vi "PRO_VerifySpecV1.vi"(6 "error in (no error)":errorcluster, 7 "Enable":bool, 8 "Results in":T7=[[{"Fill"=0.0, "Drain"=7.150000000000002, "Status"=9, "Resistor"=100.0}, {"Fill"=0.0, "Drain"=6.925000000000003, "Status"=9, "Resistor"=100.0}], [{"Fill"=7.1350000000000025, "Drain"=6.700000000000004, "Status"=9, "Resistor"=200.0}, {"Fill"=6.910000000000004, "Drain"=6.475000000000005, "Status"=9, "Resistor"=200.0}], [{"Fill"=6.685000000000004, "Drain"=6.250000000000005, "Status"=9, "Resistor"=300.0}, {"Fill"=6.460000000000004, "Drain"=6.025000000000006, "Status"=9, "Resistor"=300.0}], [{"Fill"=6.235000000000006, "Drain"=5.8000000000000025, "Status"=9, "Resistor"=400.0}, {"Fill"=6.010000000000005, "Drain"=5.59, "Status"=9, "Resistor"=400.0}], [{"Fill"=5.785000000000002, "Drain"=5.364999999999997, "Status"=9, "Resistor"=500.0}, {"Fill"=5.574999999999999, "Drain"=5.1399999999999935, "Status"=9, "Resistor"=500.0}], [{"Fill"=5.349999999999996, "Drain"=4.91499999999999, "Status"=9, "Resistor"=600.0}, {"Fill"=5.124999999999993, "Drain"=4.689999999999987, "Status"=9, "Resistor"=600.0}], [{"Fill"=4.89999999999999, "Drain"=4.464999999999983, "Status"=9, "Resistor"=700.0}, {"Fill"=4.6749999999999865, "Drain"=4.23999999999998, "Status"=9, "Resistor"=700.0}], [{"Fill"=4.449999999999983, "Drain"=4.014999999999977, "Status"=9, "Resistor"=800.0}, {"Fill"=4.22499999999998, "Drain"=3.7899999999999734, "Status"=9, "Resistor"=800.0}], [{"Fill"=3.999999999999977, "Drain"=3.56499999999997, "Status"=9, "Resistor"=900.0}, {"Fill"=3.7749999999999737, "Drain"=3.339999999999967, "Status"=9, "Resistor"=900.0}], [{"Fill"=3.5499999999999705, "Drain"=3.114999999999964, "Status"=9, "Resistor"=1000.0}, {"Fill"=3.3249999999999673, "Drain"=2.8899999999999606, "Status"=9, "Resistor"=1000.0}], [{"Fill"=3.099999999999964, "Drain"=0.0, "Status"=5, "Resistor"=1100.0}, {"Fill"=2.874999999999961, "Drain"=0.0, "Status"=5, "Resistor"=1100.0}]] {"Resistor" format="%.1f"; "Drain" format="%.3f"; "Fill" format="%.3f"}, 9 "Measure In":T6={"Ch A   Ohms"=100.0, " Ch B  Ohms"=100.0, "Level OUt"=3.672222222222213}, 10 "Specs In":T1, 11 "Switched In":bool[](array[boolean])) -> (0 "Results out":T7=[[{"Fill"=0.0, "Drain"=7.150000000000002, "Status"=9, "Resistor"=100.0}, {"Fill"=0.0, "Drain"=6.925000000000003, "Status"=9, "Resistor"=100.0}], [{"Fill"=7.1350000000000025, "Drain"=6.700000000000004, "Status"=9, "Resistor"=200.0}, {"Fill"=6.910000000000004, "Drain"=6.475000000000005, "Status"=9, "Resistor"=200.0}], [{"Fill"=6.685000000000004, "Drain"=6.250000000000005, "Status"=9, "Resistor"=300.0}, {"Fill"=6.460000000000004, "Drain"=6.025000000000006, "Status"=9, "Resistor"=300.0}], [{"Fill"=6.235000000000006, "Drain"=5.8000000000000025, "Status"=9, "Resistor"=400.0}, {"Fill"=6.010000000000005, "Drain"=5.59, "Status"=9, "Resistor"=400.0}], [{"Fill"=5.785000000000002, "Drain"=5.364999999999997, "Status"=9, "Resistor"=500.0}, {"Fill"=5.574999999999999, "Drain"=5.1399999999999935, "Status"=9, "Resistor"=500.0}], [{"Fill"=5.349999999999996, "Drain"=4.91499999999999, "Status"=9, "Resistor"=600.0}, {"Fill"=5.124999999999993, "Drain"=4.689999999999987, "Status"=9, "Resistor"=600.0}], [{"Fill"=4.89999999999999, "Drain"=4.464999999999983, "Status"=9, "Resistor"=700.0}, {"Fill"=4.6749999999999865, "Drain"=4.23999999999998, "Status"=9, "Resistor"=700.0}], [{"Fill"=4.449999999999983, "Drain"=4.014999999999977, "Status"=9, "Resistor"=800.0}, {"Fill"=4.22499999999998, "Drain"=3.7899999999999734, "Status"=9, "Resistor"=800.0}], [{"Fill"=3.999999999999977, "Drain"=3.56499999999997, "Status"=9, "Resistor"=900.0}, {"Fill"=3.7749999999999737, "Drain"=3.339999999999967, "Status"=9, "Resistor"=900.0}], [{"Fill"=3.5499999999999705, "Drain"=3.114999999999964, "Status"=9, "Resistor"=1000.0}, {"Fill"=3.3249999999999673, "Drain"=2.8899999999999606, "Status"=9, "Resistor"=1000.0}], [{"Fill"=3.099999999999964, "Drain"=0.0, "Status"=5, "Resistor"=1100.0}, {"Fill"=2.874999999999961, "Drain"=0.0, "Status"=5, "Resistor"=1100.0}]] {"Resistor" format="%.1f"; "Drain" format="%.3f"; "Fill" format="%.3f"}, 1 "Status Code":i32, 3 "Switched Out":bool[](array[boolean]), 4 "error out":errorcluster)   [LabVIEW 2024]
doc: "Compares the ChA, ChB and Level measurements to the Incexed Spec Row. Checks for R Switch Value occured in Switch Zone, The resistor level was consistand in the In Range Zone, and records the R level in ohms at the R measurement point. \n\nBuilds the Results Table."
uses:
  Control Definitions/Def Results2.ctl
  Control Definitions/Ded LUT_Status.ctl
  Control Definitions/Def PumpCtlRefs.ctl
  Control Definitions/DEF_SpecsOut.ctl
  Control Definitions/Def_ATPStatus.ctl
  Control Definitions/Def_PumpSpeed.ctl
  Control Definitions/Def Spec RNG.ctl
  Control Definitions/Def TestState.ctl
panel:
  # "ChA=0; ChB=1"
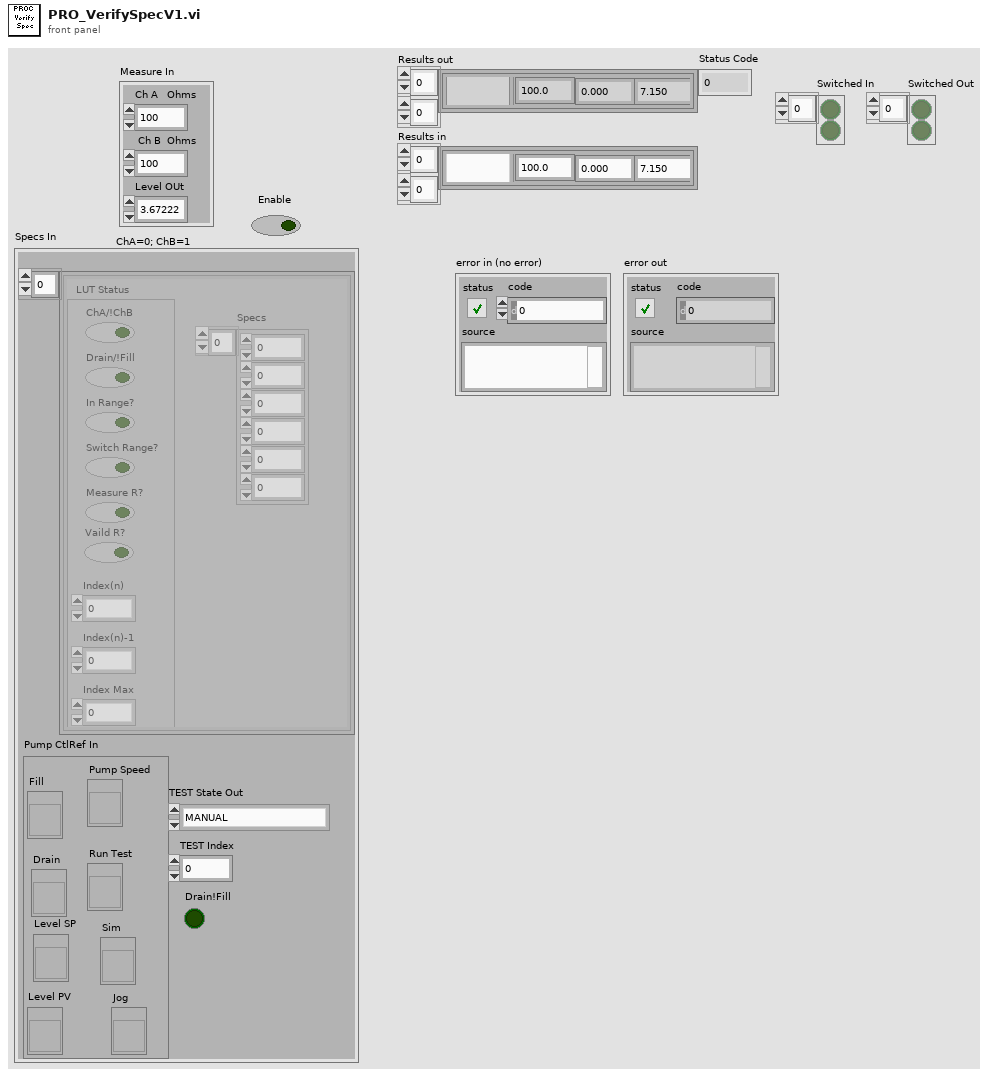
[diagram p1: front panel]
types:
  T1 = typedef "DEF_SpecsOut.ctl" = cluster{"aSpecsTable":T2[], "Pump CtlRef In":T4, "TEST State Out":T5, "TEST Index":i32, "Drain!Fill":bool}
  T2 = typedef "Def Spec RNG.ctl" = cluster{"Specs":dbl[], "LUT Status":T3}
  T3 = typedef "Ded LUT_Status.ctl" = cluster{"ChA/!ChB":bool, "Drain/!Fill":bool, "In Range?":bool, "Switch Range?":bool, "Measure R?":bool, "Vaild R?":bool, "Index(n)":i32, "Index(n)-1":i32, "Index Max":i32, "Index(n-1)":i32}
  T4 = typedef "Def PumpCtlRefs.ctl" = cluster{"Fill ":refnum<vi>, "Drain":refnum<vi>, "Level PV":refnum<vi>, "Pump Speed":refnum<vi>, "Run Test":refnum<vi>, "Sim":refnum<vi>, "Jog":refnum<vi>, "Level SP":refnum<vi>}
  T5 = typedef "Def TestState.ctl" = enum16{"MANUAL", "Start", "Pre-Fill", "Pre-Fill Measure", "Pre-Drain", "Pre-Drin Measure", "Init-Record", "Load Fill Spec", "Filling Hi", "Wait1", "Record Fill", "Load Drain Spec", "Draining Lo", "Wait2", "Record Drain", "Empty", "Done"}
  T6 = cluster{"Ch A   Ohms":dbl, " Ch B  Ohms":dbl, "Level OUt":dbl}
  T7 = typedef "Def Results2.ctl" = cluster{"Fill":dbl, "Drain":dbl, "Status":T8, "Resistor":dbl}[][]
  T8 = typedef "Def_ATPStatus.ctl" = i16
  T9 = cluster{"Fill":dbl, "Drain":dbl, "Status":T8, "Resistor":dbl}
  T10 = cluster{"Fill":dbl, "Drain":dbl, "Status":i16, "Resistor":dbl}[]
  T11 = typedef "Def_LevelSwitched.ctl" = cluster{"Switched":bool, "Level OUt":dbl, "Double Err":bool}
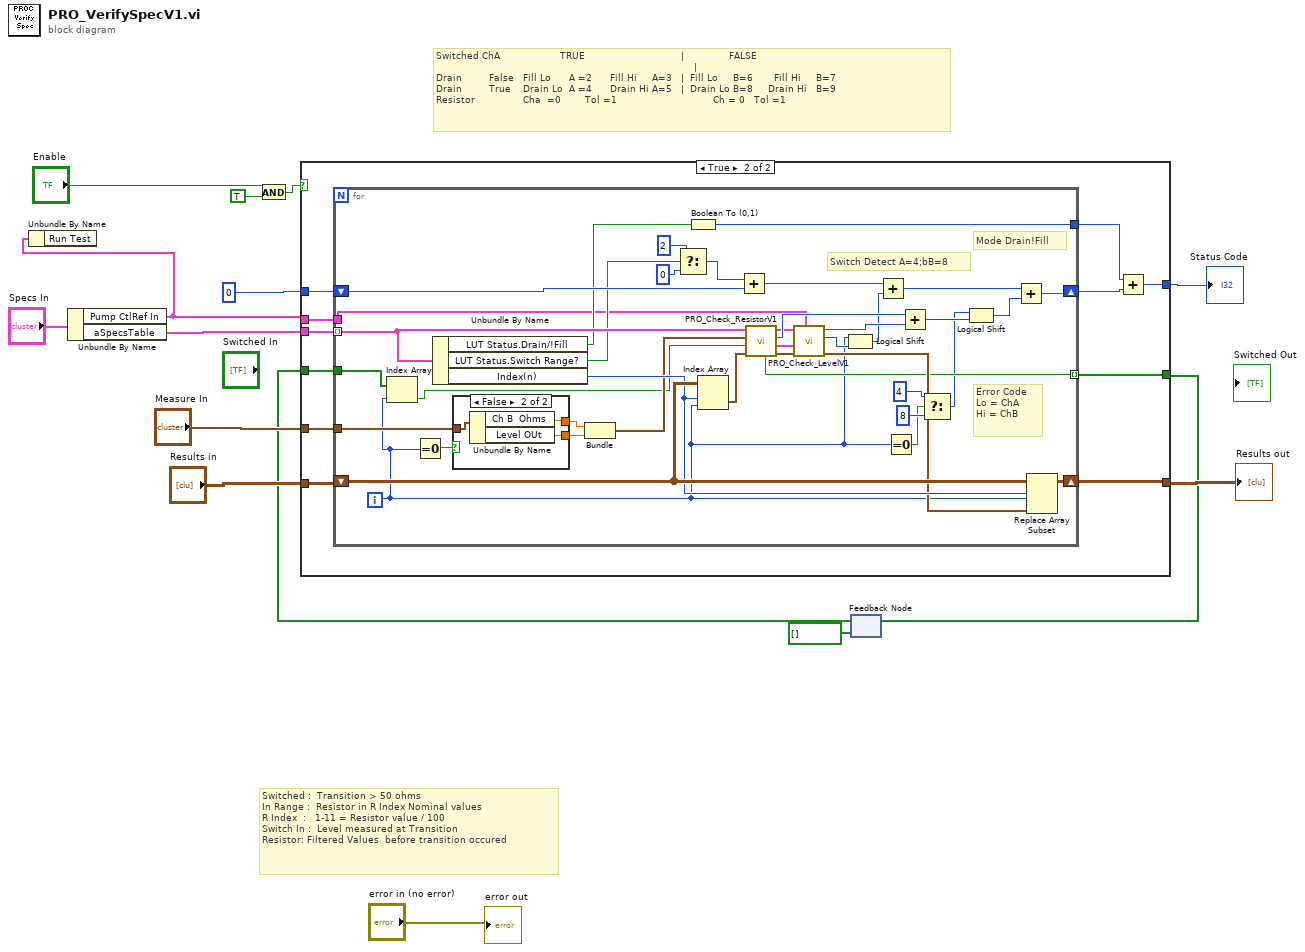
[diagram p0: block diagram]
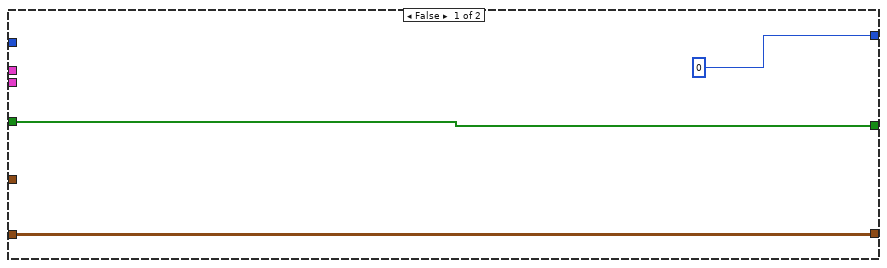
[diagram p2: hidden frame]
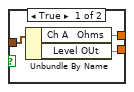
[diagram p3: hidden frame]
diagram:
  # "Switched ChA                    TRUE                                |               FALSE\n                                                                                      |\nDrain         False   Fill Lo      A =2      Fill Hi     A=3   |  Fill Lo     B=6       Fill Hi     B=7\nDrain         True    Drain Lo  A =4      Drain Hi A=5   |  Drain Lo B=8     Drain Hi   B=9 \nResistor                Cha  =0        Tol =1                                Ch = 0   Tol =1"
  # "Switched :  Transition > 50 ohms\nIn Range :  Resistor in R Index Nominal values\nR Index  :   1-11 = Resistor value / 100\nSwitch In :  Level measured at Transition\nResistor: Filtered Values  before transition occured"
  n1 = Unbundle By Name("Specs In") -> ("Pump CtlRef In"=w7:T4, "aSpecsTable"=w8:T2[])
  n2 = Unbundle By Name(w7) -> ()  [unwired: 1 out]
  n3 = And(x="Enable", y=TRUE) -> (x .and. y?=w6:bool)
  n4 = feedback #1(bool[] []) -> (w3:bool[])
  n5 = case shown="True" w6 {
    tunnel: w8 -> [_ w29]
    tunnel: "Results in" -> [w17 w28]
    tunnel: [w17 w27] -> w13
    tunnel: 0 -> [_ w26]
    tunnel: [0 w22] -> w11
    tunnel: "Measure In" -> [_ w25]
    tunnel: w3 -> [w16 w23]
    tunnel: [w16 w24] -> w4
    tunnel: w7 -> [_ w19]
    frame False {
    }
    frame True {
      n6 = for {
        tunnel: w29 -> [w62] mode=indexing
        shift-right: [w52] -> w27
        shift-left: w28 -> [w68]
        shift-right: [w49] -> w21
        shift-left: w26 -> [w43]
        tunnel: w25 -> [w65]
        tunnel: [w51] -> w24 mode=indexing
        tunnel: w23 -> [w55]
        tunnel: [w34] -> w20
        tunnel: w19 -> [w30]
        i -> [w40]
        # "Switch Detect A=4;bB=8"
        # "Mode Drain!Fill"
        # "Error Code\nLo = ChA\nHi = ChB"
        n7 = Index Array(array=w55, index=w40) -> (element=w31:bool)
        n8 = Equal To 0?(x=w40) -> (x = 0?=w64:bool)
        n9 = Unbundle By Name(w62) -> ("LUT Status.Drain/!Fill"=w36:bool, "LUT Status.Switch Range?"=w33:bool, "Index(n)"=w67:i32)
        n10 = case shown="False" w64 {
          tunnel: w65 -> [w71 w74]
          tunnel: [w70 w73] -> w63
          tunnel: [w69 w72] -> w32
          frame True {
            n11 = Unbundle By Name(w71) -> ("Ch A   Ohms"=w70:dbl, "Level OUt"=w69:dbl)
          }
          frame False {
            n12 = Unbundle By Name(w74) -> ("Ch B  Ohms"=w73:dbl, "Level OUt"=w72:dbl)
          }
        }
        n13 = Bundle("Ch B  Ohms"=w63, "Level OUt"=w32) -> (w61:cluster{" Ch B  Ohms":dbl, "Level OUt":dbl})  [unwired: 1 in]
        n14 = Select(t=2, s=w33, f=0) -> (s? t:f=w35:i32)
        n15 = Boolean To (0,1)(Boolean=w36) -> (0, 1=w34:i16)
        n16 = Index Array(array=w68, index (row)=w67, index (col)=w40) -> (element=w60:T9)
        n17 = Add(x=w35, y=w43) -> (x+y=w42:i32)
        n18 = call "PRO_Check_ResistorV1.vi"("Results IN"=w60, "Switched In"=w31, "Inputs"=w61, "ChA Spec RNG In"=w62) -> ("results out"=w58:T10, "Level Out"=w57:T11, "Err Num"=w59:i32, "ChA Spec RNG Out"=w56:T2, "Switched Out"=w51:bool)  [unwired: 3 in]
        n19 = call "PRO_Check_LevelV1.vi"(7:w30, "Results In"=w58, "Level In"=w57, "ChA Spec RNG In"=w56) -> ("Results Out"=w66:T10, "Switched Code"=w41:i32, "Err Num"=w45:i32)  [unwired: 4 in, 1 out]
        n20 = Logical Shift(y=w40, x=w41) -> (x << y=w44:i32)
        n21 = Add(x=w42, y=w44) -> (x+y=w37:i32)
        n22 = Equal To 0?(x=w40) -> (x = 0?=w50:bool)
        n23 = Add(x=w59, y=w45) -> (x+y=w39:i32)
        n24 = Select(t=4, s=w50, f=8 ("x")) -> (s? t:f=w38:i32)
        n25 = Logical Shift(y=w38, x=w39) -> (x << y=w46:i32)
        n26 = Add(x=w37, y=w46) -> (x+y=w49:i32)
        n27 = Replace Array Subset(array=w68, new element=w66, index (row)=w67, index (col)=w40) -> (w52:T7)
      }
      n28 = Add(x=w20, y=w21) -> (x+y=w22:i32)
    }
  }
  "Results out" <- w13
  "Status Code" <- w11
  n29 = feedback-in #1(w4) -> ()
  "error out" <- "error in (no error)"
